vi "UMLEditor RoundToNearestN.vi"(1 "N":dbl format="%.2f", 2 "IN":dbl format="%.2f") -> (0 "UT":dbl format="%.2f")   [LabVIEW 2014]
doc: "Round the IN-number to nearest N."
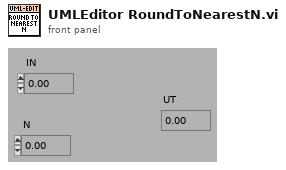
[diagram p1: front panel]
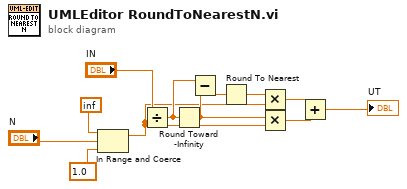
[diagram p0: block diagram]
diagram:
  n1 = In Range and Coerce(upper limit=inf, x="N", lower limit=1.0) -> (coerced(x)=w1:dbl)  [unwired: 1 out]
  n2 = Divide(x="IN", y=w1) -> (x/y=w7:dbl)
  n3 = Round Toward -Infinity(1:w7) -> (0:w6:dbl)
  n4 = Subtract(x=w7, y=w6) -> (x-y=w5:dbl)
  n5 = Round To Nearest(number=w5) -> (nearest integer value=w10:dbl)
  n6 = Multiply(x=w10, y=w1) -> (x*y=w9:dbl)
  n7 = Multiply(x=w6, y=w1) -> (x*y=w12:dbl)
  n8 = Add(x=w9, y=w12) -> (x+y=→"UT":dbl)
